vi "VI Tree.vi"   [LabVIEW 2012, in "Datron D4xxx.lvlib"]
doc: "This is the instrument driver for the <INSTRUMENT NAME>. The VI Tree displays all the user-callable VIs of the instrument driver in an organized table."
uses:
  Datron D4xxx.lvlib
panel:
  # "(c) 2007 <Enter Company Name Here>.  ALL RIGHTS RESERVED."
  # "SEE DIAGRAM\nFOR VI TREE."
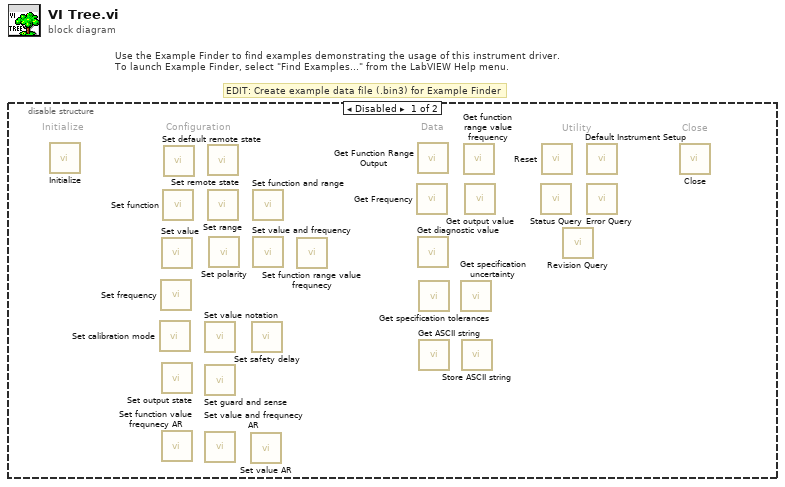
[diagram p0: block diagram]
diagram:
  # "EDIT: Create example data file (.bin3) for Example Finder"
  # "Use the Example Finder to find examples demonstrating the usage of this instrument driver.\nTo launch Example Finder, select \"Find Examples...\" from the LabVIEW Help menu."
  n1 = disable-structure shown="Disabled" {
    frame Disabled {
      # "Configuration"
      # "Utility"
      # "Data"
      # "Close"
      # "Initialize"
      n2 = call "Initialize.vi"() -> ()  [unwired: 10 in, 2 out]
      n3 = call "Set calibration mode.vi"() -> ()  [unwired: 10 in, 2 out]
      n4 = call "Set frequency.vi"() -> ()  [unwired: 9 in, 3 out]
      n5 = call "Set value.vi"() -> ()  [unwired: 9 in, 3 out]
      n6 = call "Set output state.vi"() -> ()  [unwired: 10 in, 2 out]
      n7 = call "Set function value frequnecy AR.vi"() -> ()  [unwired: 9 in, 3 out]
      n8 = call "Set function.vi"() -> ()  [unwired: 10 in, 2 out]
      n9 = call "Set default remote state.vi"() -> ()  [unwired: 10 in, 2 out]
      n10 = call "Set value notation.vi"() -> ()  [unwired: 10 in, 2 out]
      n11 = call "Set guard and sense.vi"() -> ()  [unwired: 8 in, 4 out]
      n12 = call "Set value and frequnecy AR.vi"() -> ()  [unwired: 9 in, 3 out]
      n13 = call "Set remote state.vi"() -> ()  [unwired: 10 in, 2 out]
      n14 = call "Set range.vi"() -> ()  [unwired: 10 in, 2 out]
      n15 = call "Set polarity.vi"() -> ()  [unwired: 10 in, 2 out]
      n16 = call "Set value AR.vi"() -> ()  [unwired: 9 in, 3 out]
      n17 = call "Set safety delay.vi"() -> ()  [unwired: 10 in, 2 out]
      n18 = call "Set function and range.vi"() -> ()  [unwired: 10 in, 2 out]
      n19 = call "Set value and frequency.vi"() -> ()  [unwired: 9 in, 3 out]
      n20 = call "Set function range value frequnecy.vi"() -> ()  [unwired: 9 in, 3 out]
      n21 = call "Get Frequency.vi"() -> ()  [unwired: 9 in, 3 out]
      n22 = call "Get Function Range Output.vi"() -> ()  [unwired: 4 in, 8 out]
      n23 = call "Get diagnostic value.vi"() -> ()  [unwired: 8 in, 4 out]
      n24 = call "Get specification tolerances.vi"() -> ()  [unwired: 4 in, 8 out]
      n25 = call "Get ASCII string.vi"() -> ()  [unwired: 9 in, 3 out]
      n26 = call "Get specification uncertainty.vi"() -> ()  [unwired: 4 in, 8 out]
      n27 = call "Store ASCII string.vi"() -> ()  [unwired: 10 in, 2 out]
      n28 = call "Get function range value frequency.vi"() -> ()  [unwired: 4 in, 8 out]
      n29 = call "Get output value.vi"() -> ()  [unwired: 9 in, 3 out]
      n30 = call "Status Query.vi"() -> ()  [unwired: 7 in, 9 out]
      n31 = call "Reset.vi"() -> ()  [unwired: 10 in, 2 out]
      n32 = call "Revision Query.vi"() -> ()  [unwired: 9 in, 3 out]
      n33 = call "Default Instrument Setup.vi"() -> ()  [unwired: 10 in, 2 out]
      n34 = call "Error Query.vi"() -> ()  [unwired: 8 in, 4 out]
      n35 = call "Close.vi"() -> ()  [unwired: 11 in, 1 out]
    }
    frame Enabled {
    }
  }
